vi "closeSession.vi"(2 "error in (no error)":errorcluster, 3 "FrequencyCounter in":refnum<class "FrequencyCounter.lvclass">) -> (0 "error out":errorcluster, 1 "FrequencyCounter out":refnum<class "FrequencyCounter.lvclass">)   [LabVIEW 2009, in "Hardware.lvlib" / "frequencyCounters.lvlib" / "FrequencyCounter.lvclass"]
uses:
  FrequencyCounter.lvclass
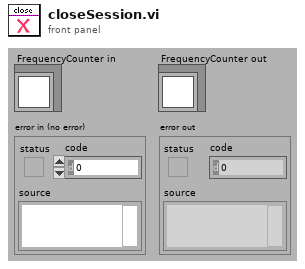
[diagram p1: front panel]
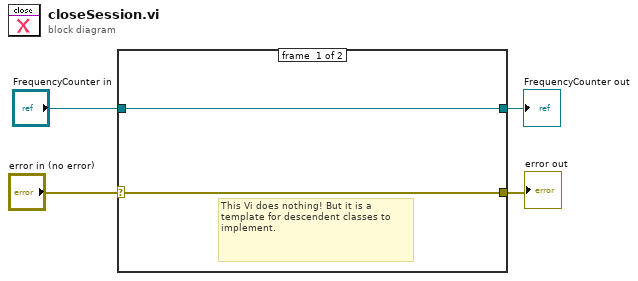
[diagram p0: block diagram]
diagram:
  n1 = case shown="No Error" "error in (no error)" {
    selector: "error in (no error)" -> [w5 w8]
    tunnel: [w5 w8] -> w3
    tunnel: [w6 w7] -> w1
    tunnel: "FrequencyCounter in" -> [w6 w7]
    frame #0 {
      # "This Vi does nothing! But it is a template for descendent classes to implement."
    }
    frame #1 {
    }
  }
  "error out" <- w3
  "FrequencyCounter out" <- w1
